vi "5 x Lesen Grenzwerte.vi"(5 "Datenfluss (in)":bool, 8 "Fehler (Eingang, kein Fehler)":errorcluster, 9 "Factorysettings":path, 11 "appended path":path) -> (0 "Fehler (Ausgang)":errorcluster, 3 "Anlagen-Grenzwerte Anzeige":T1 {"Heizleitung zu FT-IR:"."Abschalt-Max" format="%#_5g"; "Heizleitung zu FT-IR:"."Abschalt-Min" format="%#_5g"; "Heizleitung zu FT-IR:"."Warn-Max" format="%#_5g"; "Heizleitung zu FT-IR:"."Warn-Min" format="%#_5g"; "Heizleitung zu FT-IR:"."Sollwert" format="%#_5g"; "Heizleitung zu FT-IR:"."Regler" items=["inaktiv", "aktiv"]; "Druck Kalter Block:"."Abschalt-Max" format="%#_5g"; "Druck Kalter Block:"."Abschalt-Min" format="%#_5g"; "Druck Kalter Block:"."Warn-Max" format="%#_5g"; "Druck Kalter Block:"."Warn-Min" format="%#_5g"; "Druck Kalter Block:"."Sollwert" format="%#_5g"; "Druck Kalter Block:"."Regler" items=["inaktiv", "aktiv"]; "Durchfluss CalGas:"."Abschalt-Max" format="%#_5g"; "Durchfluss CalGas:"."Abschalt-Min" format="%#_5g"; "Durchfluss CalGas:"."Warn-Max" format="%#_5g"; "Durchfluss CalGas:"."Warn-Min" format="%#_5g"; "Durchfluss CalGas:"."Sollwert" format="%#_5g"; "Durchfluss CalGas:"."Regler" items=["inaktiv", "aktiv"]; "Heizleitung Extern SP2:"."Abschalt-Max" format="%#_5g"; "Heizleitung Extern SP2:"."Abschalt-Min" format="%#_5g"; "Heizleitung Extern SP2:"."Warn-Max" format="%#_5g"; "Heizleitung Extern SP2:"."Warn-Min" format="%#_5g"; "Heizleitung Extern SP2:"."Sollwert" format="%#_5g"; "Heizleitung Extern SP2:"."Regler" items=["inaktiv", "aktiv"]; "Gaskühler:"."Abschalt-Max" format="%#_5g"; "Gaskühler:"."Abschalt-Min" format="%#_5g"; "Gaskühler:"."Warn-Max" format="%#_5g"; "Gaskühler:"."Warn-Min" format="%#_5g"; "Gaskühler:"."Sollwert" format="%#_5g"; "Gaskühler:"."Regler" items=["inaktiv", "aktiv"]; "Heizleitung Extern SP1:"."Abschalt-Max" format="%#_5g"; "Heizleitung Extern SP1:"."Abschalt-Min" format="%#_5g"; "Heizleitung Extern SP1:"."Warn-Max" format="%#_5g"; "Heizleitung Extern SP1:"."Warn-Min" format="%#_5g"; "Heizleitung Extern SP1:"."Sollwert" format="%#_5g"; "Heizleitung Extern SP1:"."Regler" items=["inaktiv", "aktiv"]; "Schaltschranktemperatur:"."Abschalt-Max" format="%#_5g"; "Schaltschranktemperatur:"."Abschalt-Min" format="%#_5g"; "Schaltschranktemperatur:"."Warn-Max" format="%#_5g"; "Schaltschranktemperatur:"."Warn-Min" format="%#_5g"; "Schaltschranktemperatur:"."Sollwert" format="%#_5g"; "Schaltschranktemperatur:"."Regler" items=["inaktiv", "aktiv"]; "FT-IR Heizung Messzelle:"."Abschalt-Max" format="%#_5g"; "FT-IR Heizung Messzelle:"."Abschalt-Min" format="%#_5g"; "FT-IR Heizung Messzelle:"."Warn-Max" format="%#_5g"; "FT-IR Heizung Messzelle:"."Warn-Min" format="%#_5g"; "FT-IR Heizung Messzelle:"."Sollwert" format="%#_5g"; "FT-IR Heizung Messzelle:"."Regler" items=["inaktiv", "aktiv"]; "Heizung Pumpe:"."Abschalt-Max" format="%#_5g"; "Heizung Pumpe:"."Abschalt-Min" format="%#_5g"; "Heizung Pumpe:"."Warn-Max" format="%#_5g"; "Heizung Pumpe:"."Warn-Min" format="%#_5g"; "Heizung Pumpe:"."Sollwert" format="%#_5g"; "Heizung Pumpe:"."Regler" items=["inaktiv", "aktiv"]; "Heizung Filterblock:"."Abschalt-Max" format="%#_5g"; "Heizung Filterblock:"."Abschalt-Min" format="%#_5g"; "Heizung Filterblock:"."Warn-Max" format="%#_5g"; "Heizung Filterblock:"."Warn-Min" format="%#_5g"; "Heizung Filterblock:"."Sollwert" format="%#_5g"; "Heizung Filterblock:"."Regler" items=["inaktiv", "aktiv"]; "Heizleitungen intern:"."Abschalt-Max" format="%#_5g"; "Heizleitungen intern:"."Abschalt-Min" format="%#_5g"; "Heizleitungen intern:"."Warn-Max" format="%#_5g"; "Heizleitungen intern:"."Warn-Min" format="%#_5g"; "Heizleitungen intern:"."Sollwert" format="%#_5g"; "Heizleitungen intern:"."Regler" items=["inaktiv", "aktiv"]; "Druck Ausgang:"."Abschalt-Max" format="%#_5g"; "Druck Ausgang:"."Abschalt-Min" format="%#_5g"; "Druck Ausgang:"."Warn-Max" format="%#_5g"; "Druck Ausgang:"."Warn-Min" format="%#_5g"; "Druck Ausgang:"."Sollwert" format="%#_5g"; "Druck Ausgang:"."Regler" items=["inaktiv", "aktiv"]; "Durchfluss FT-IR:"."Abschalt-Max" format="%#_5g"; "Durchfluss FT-IR:"."Abschalt-Min" format="%#_5g"; "Durchfluss FT-IR:"."Warn-Max" format="%#_5g"; "Durchfluss FT-IR:"."Warn-Min" format="%#_5g"; "Durchfluss FT-IR:"."Sollwert" format="%#_5g"; "Durchfluss FT-IR:"."Regler" items=["inaktiv", "aktiv"]; "Eingangsdruck FT-IR:"."Abschalt-Max" format="%#_5g"; "Eingangsdruck FT-IR:"."Abschalt-Min" format="%#_5g"; "Eingangsdruck FT-IR:"."Warn-Max" format="%#_5g"; "Eingangsdruck FT-IR:"."Warn-Min" format="%#_5g"; "Eingangsdruck FT-IR:"."Sollwert" format="%#_5g"; "Eingangsdruck FT-IR:"."Regler" items=["inaktiv", "aktiv"]}, 4 "Datenfluss (out)":bool)   [LabVIEW 2020, in "Konfig-Dateien.lvlib"]
uses:
  Konfig-Dateien.lvlib
  Seiten/Anlagengrenzwerte/Anlagen-Grenzwerte Anzeige.ctl
  Seiten/Anlagengrenzwerte/Anlagen-Parameter Anzeige.ctl
  SysLog/SysLog Interface cRIO.ctl
  Seiten/Anlagengrenzwerte/Anlagengrenzwerte.lvlib
  SysLog/SysLog_cRIO.lvlib
panel:
  # "°C"
  # "°C"
  # "°C"
  # "mbar"
  # "mbar"
  # "mbar"
  # "l/min"
  # "l/min"
  # "l/min"
  # "°C"
  # "°C"
  # "°C"
  # "°C"
  # "°C"
  # "°C"
  # "°C"
  # "°C"
  # "°C"
  # "°C"
  # "°C"
  # "°C"
  # "°C"
  # "°C"
  # "°C"
  # "°C"
  # "°C"
  # "°C"
  # "°C"
  # "°C"
  # "°C"
  # "°C"
  # "°C"
  # "°C"
  # "mbar"
  # "mbar"
  # "mbar"
  # "l/min"
  # "l/min"
  # "l/min"
  # "atm"
  # "atm"
  # "atm"
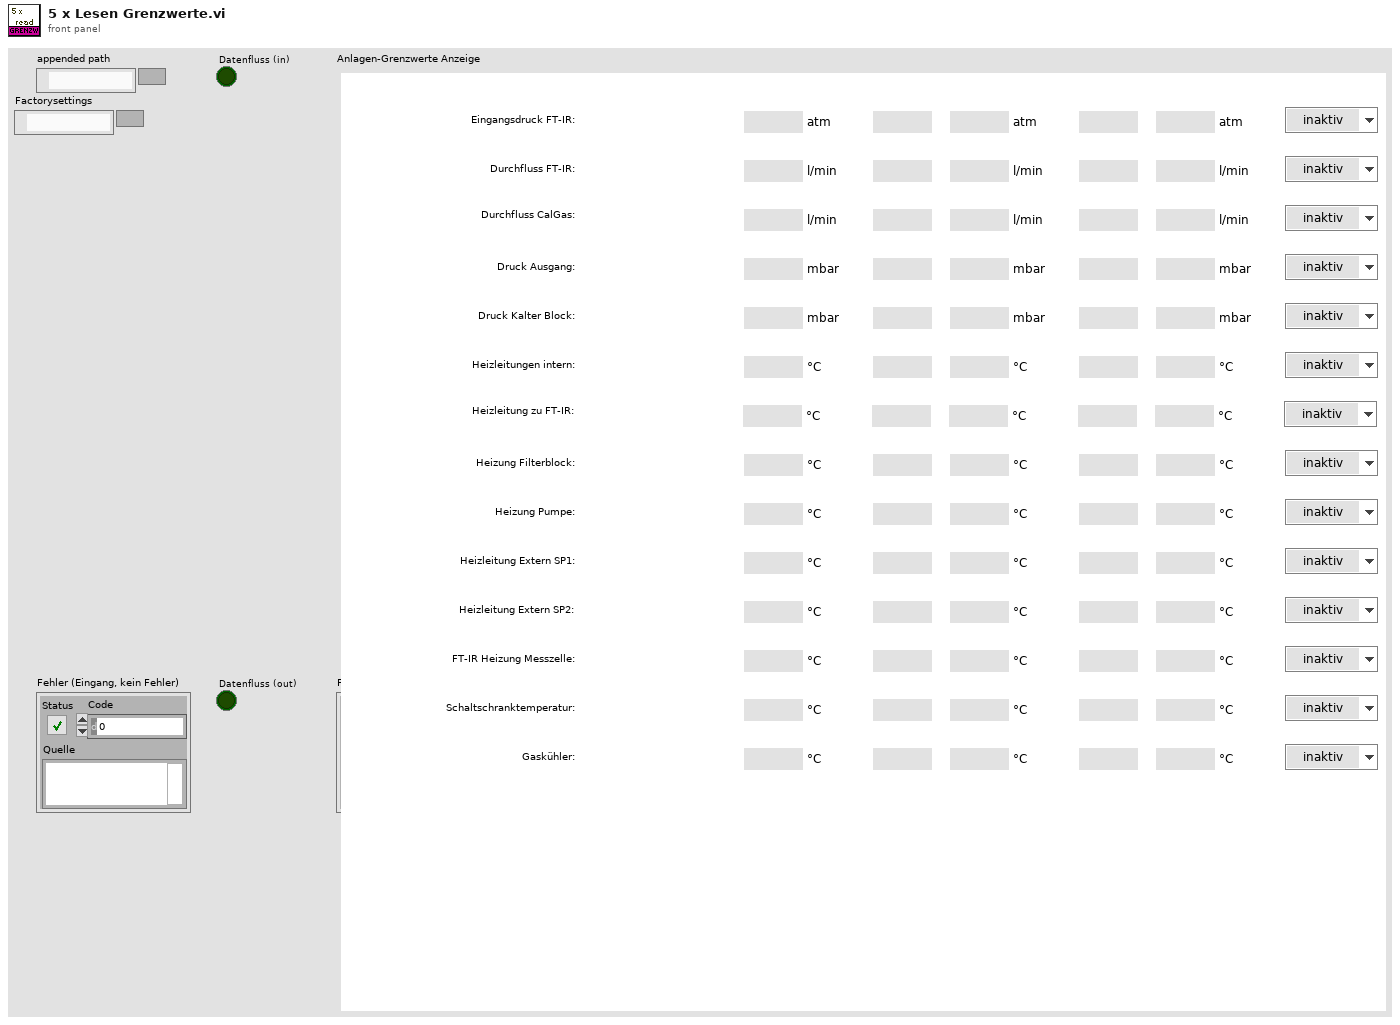
[diagram p1: front panel]
types:
  T1 = typedef "Anlagengrenzwerte.lvlib/Anlagen-Grenzwerte Anzeige.ctl" = cluster{"Eingangsdruck FT-IR:":T2, "Durchfluss FT-IR:":T2, "Durchfluss CalGas:":T2, "Druck Ausgang:":T2, "Druck Kalter Block:":T2, "Heizleitungen intern:":T2, "Heizleitung zu FT-IR:":T2, "Heizung Filterblock:":T2, "Heizung Pumpe:":T2, "Heizleitung Extern SP1:":T2, "Heizleitung Extern SP2:":T2, "FT-IR Heizung Messzelle:":T2, "Schaltschranktemperatur:":T2, "Gaskühler:":T2}
  T2 = typedef "Anlagengrenzwerte.lvlib/Anlagen-Parameter Anzeige.ctl" = cluster{"Sollwert":sgl, "Warn-Min":sgl, "Warn-Max":sgl, "Abschalt-Min":sgl, "Abschalt-Max":sgl, "Regler":u16}
  T3 = typedef "SysLog_cRIO.lvlib/SysLog Interface cRIO.ctl" = cluster{"FehlermeldungsCode":i32, "ErfolgsmeldungsCode":i32, "ParameterListenString":string, "intern":bool}
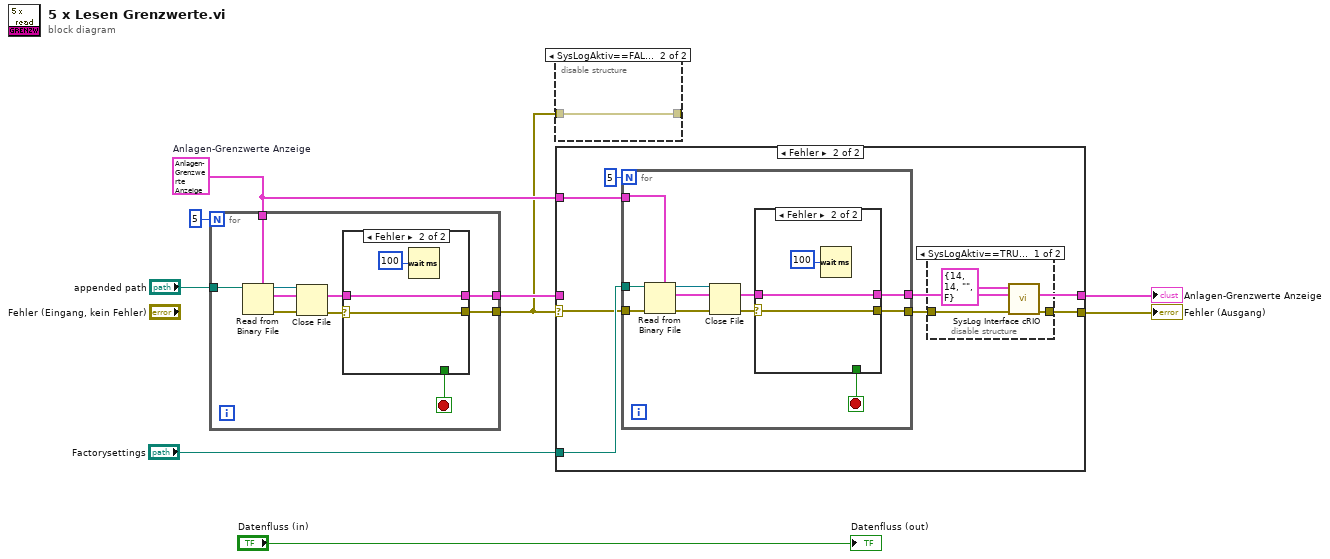
[diagram p0: block diagram]
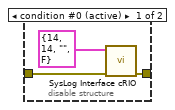
[diagram p2: hidden frame]
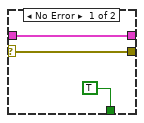
[diagram p5: hidden frame]
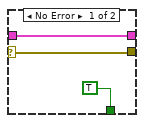
[diagram p6: hidden frame]
diagram:
  w2 = T1 {"Eingangsdruck FT-IR:"={"Sollwert"=0.0, "Warn-Min"=0.0, "Warn-Max"=0.0, "Abschalt-Min"=0.0, "Abschalt-Max"=0.0, "Regler"=0}, "Durchfluss FT-IR:"={"Sollwert"=0.0, "Warn-Min"=0.0, "Warn-Max"=0.0, "Abschalt-Min"=0.0, "Abschalt-Max"=0.0, "Regler"=0}, "Durchfluss CalGas:"={"Sollwert"=0.0, "Warn-Min"=0.0, "Warn-Max"=0.0, "Abschalt-Min"=0.0, "Abschalt-Max"=0.0, "Regler"=0}, "Druck Ausgang:"={"Sollwert"=0.0, "Warn-Min"=0.0, "Warn-Max"=0.0, "Abschalt-Min"=0.0, "Abschalt-Max"=0.0, "Regler"=0}, "Druck Kalter Block:"={"Sollwert"=0.0, "Warn-Min"=0.0, "Warn-Max"=0.0, "Abschalt-Min"=0.0, "Abschalt-Max"=0.0, "Regler"=0}, "Heizleitungen intern:"={"Sollwert"=0.0, "Warn-Min"=0.0, "Warn-Max"=0.0, "Abschalt-Min"=0.0, "Abschalt-Max"=0.0, "Regler"=0}, "Heizleitung zu FT-IR:"={"Sollwert"=0.0, "Warn-Min"=0.0, "Warn-Max"=0.0, "Abschalt-Min"=0.0, "Abschalt-Max"=0.0, "Regler"=0}, "Heizung Filterblock:"={"Sollwert"=0.0, "Warn-Min"=0.0, "Warn-Max"=0.0, "Abschalt-Min"=0.0, "Abschalt-Max"=0.0, "Regler"=0}, "Heizung Pumpe:"={"Sollwert"=0.0, "Warn-Min"=0.0, "Warn-Max"=0.0, "Abschalt-Min"=0.0, "Abschalt-Max"=0.0, "Regler"=0}, "Heizleitung Extern SP1:"={"Sollwert"=0.0, "Warn-Min"=0.0, "Warn-Max"=0.0, "Abschalt-Min"=0.0, "Abschalt-Max"=0.0, "Regler"=0}, "Heizleitung Extern SP2:"={"Sollwert"=0.0, "Warn-Min"=0.0, "Warn-Max"=0.0, "Abschalt-Min"=0.0, "Abschalt-Max"=0.0, "Regler"=0}, "FT-IR Heizung Messzelle:"={"Sollwert"=0.0, "Warn-Min"=0.0, "Warn-Max"=0.0, "Abschalt-Min"=0.0, "Abschalt-Max"=0.0, "Regler"=0}, "Schaltschranktemperatur:"={"Sollwert"=0.0, "Warn-Min"=0.0, "Warn-Max"=0.0, "Abschalt-Min"=0.0, "Abschalt-Max"=0.0, "Regler"=0}, "Gaskühler:"={"Sollwert"=0.0, "Warn-Min"=0.0, "Warn-Max"=0.0, "Abschalt-Min"=0.0, "Abschalt-Max"=0.0, "Regler"=0}}  # Anlagen-Grenzwerte Anzeige
  n1 = for {
    N: 5 -> [_]
    tunnel: [w15] -> w6
    tunnel: "appended path" -> [w18]
    tunnel: [w11] -> w1
    tunnel: w2 -> [w14]
    stop <- w17 stop-if-true
    n2 = Read from Binary File(5:w14, 11:w18) -> (0:w12:errorcluster, 2:w16:T1, 3:w13:refnum<file>)  [unwired: 4 in, 1 out]
    n3 = Close File(refnum=w13, error in=w12) -> (error out=w10:errorcluster)  [unwired: 1 out]
    n4 = case shown="Fehler" w10 {
      selector: w10 -> [w19 w22]
      tunnel: [TRUE _] -> w17
      tunnel: w16 -> [w20 w24]
      tunnel: [w20 w24] -> w15
      tunnel: [w19 w22] -> w11
      frame No Error {
      }
      frame Error {
        n5 = Wait (ms)(milliseconds to wait=u32 100 ("Zu wartende ms")) -> ()  [unwired: 1 out]
      }
    }
  }
  n6 = disable-structure shown="SysLogAktiv==FALSE, Standard" {
    disable-tunnel: w1 -> [w26 w28]
    disable-tunnel: [w25 w28] -> _
    frame condition #0 (active) {
      n7 = call "SysLog Interface cRIO.vi"("Fehler (in)"=w26, "Cluster (in)"=T3 {"FehlermeldungsCode"=14, "ErfolgsmeldungsCode"=14, "ParameterListenString"="", "intern"=FALSE}) -> ("Fehler (Ausgang)"=w25:errorcluster)  [unwired: 9 in]
    }
    frame condition #1 {
    }
  }
  n8 = case shown="Fehler" w1 {
    selector: w1 -> [w29 w34]
    tunnel: w6 -> [w30 _]
    tunnel: [w30 w35] -> w5
    tunnel: "Factorysettings" -> [_ w36]
    tunnel: [w29 w32] -> w3
    tunnel: w2 -> [_ w31]
    frame No Error {
    }
    frame Error {
      n9 = for {
        N: 5 -> [_]
        tunnel: [w46] -> w35
        tunnel: w36 -> [w50]
        tunnel: w34 -> [w45]
        tunnel: [w42] -> w33
        tunnel: w31 -> [w44]
        stop <- w48 stop-if-true
        n10 = Read from Binary File(5:w44, 8:w45, 11:w50) -> (0:w49:errorcluster, 2:w47:T1, 3:w43:refnum<file>)  [unwired: 3 in, 1 out]
        n11 = Close File(refnum=w43) -> ()  [unwired: 1 in, 2 out]
        n12 = case shown="Fehler" w49 {
          selector: w49 -> [w51 w55]
          tunnel: [TRUE _] -> w48
          tunnel: w47 -> [w52 w56]
          tunnel: [w52 w56] -> w46
          tunnel: [w51 w55] -> w42
          frame No Error {
          }
          frame Error {
            n13 = Wait (ms)(milliseconds to wait=u32 100 ("Zu wartende ms")) -> ()  [unwired: 1 out]
          }
        }
      }
      n14 = disable-structure shown="SysLogAktiv==TRUE" {
        disable-tunnel: w33 -> [w39 w41]
        disable-tunnel: [w38 w41] -> w32
        frame condition #0 (active) {
          n15 = call "SysLog Interface cRIO.vi"("Fehler (in)"=w39, "Cluster (in)"=T3 {"FehlermeldungsCode"=14, "ErfolgsmeldungsCode"=14, "ParameterListenString"="", "intern"=FALSE}) -> ("Fehler (Ausgang)"=w38:errorcluster)  [unwired: 9 in]
        }
        frame condition #1 {
        }
      }
    }
  }
  "Fehler (Ausgang)" <- w3
  "Anlagen-Grenzwerte Anzeige" <- w5
  "Datenfluss (out)" <- "Datenfluss (in)"
